vi "readArmPotValues.vi"(11 "set":bool) -> (3 "Normalized Value":dbl format="%#.5f")   [LabVIEW 2018]
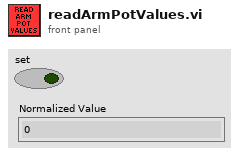
[diagram p1: front panel]
types:
  T1 = enum16{"open", "replace", "create", "open or create", "replace or create", "replace or create with confirmation"}
  T2 = typedef "WPI_PotentiometerDevRef.ctl" = cluster{"DevStatus":errorcluster, "Analog Channel":T3, "Invert Output":bool}
  T3 = typedef "FPGA_AIChannel.ctl" = enum8{"AI 0", "AI 1", "AI 2", "AI 3", "AI MXP 0", "AI MXP 1", "AI MXP 2", "AI MXP 3", "Invalid"}
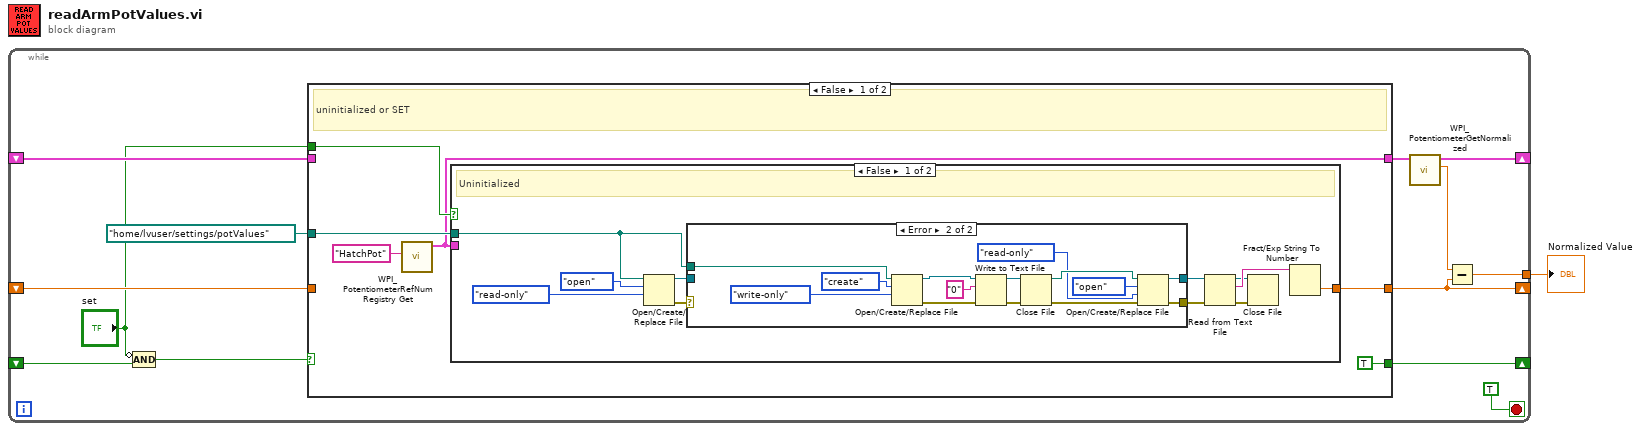
[diagram p0: block diagram]
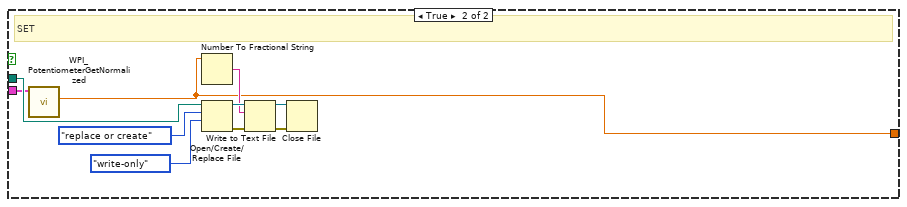
[diagram p3: hidden frame]
diagram:
  n1 = while {
    shift-right: [w14] -> _
    shift-left: _ -> [w13]
    shift-right: [w10] -> _
    shift-left: _ -> [w12]
    tunnel: [w7] -> w1
    shift-right: [w6] -> _
    shift-left: _ -> [w5]
    stop <- TRUE stop-if-true
    n2 = Compound Arithmetic op=AND(invert "set", w13) -> (w4:bool)
    n3 = case shown="False" w4 {
      selector: w4 -> [_ w60]
      tunnel: [TRUE w60] -> w14
      tunnel: [w15 w59] -> w11
      tunnel: w12 -> [_ w59]
      tunnel: [w18 w58] -> w6
      tunnel: w5 -> [_ w58]
      tunnel: "set" -> [w17 _]
      tunnel: path "/home/lvuser/settings/potValues" ("file path (use dialog)") -> [w16 _]
      frame False {
        # "uninitialized or SET"
        n4 = call <vilib>:"WPI_PotentiometerRefNum Registry Get.vi"("refnum name"="HatchPot") -> ("PotDevRef"=w15:T2)  [unwired: 9 in, 1 out]
        n5 = case shown="False" w17 {
          tunnel: [w24 w49] -> w18
          tunnel: w16 -> [w23 w50]
          tunnel: w15 -> [_ w48]
          frame False {
            # "Uninitialized"
            n6 = Open/Create/Replace File(file path (use dialog)=w23, operation (0:open)=T1."open", access (0:read/write)=enum16{"read/write", "read-only", "write-only"}."read-only") -> (refnum out=w28:refnum<file>, error out=w29:errorcluster)  [unwired: 3 in, 1 out]
            n7 = case shown="Error" w29 {
              selector: w29 -> [w33 _]
              tunnel: w28 -> [w32 _]
              tunnel: w23 -> [_ w47]
              tunnel: [w33 w34] -> w27
              tunnel: [w32 w35] -> w26
              frame No Error {
              }
              frame Error {
                n8 = Open/Create/Replace File(file path (use dialog)=w47, operation (0:open)=T1."create", access (0:read/write)=enum16{"read/write", "read-only", "write-only"}."write-only") -> (refnum out=w43:refnum<file>, error out=w44:errorcluster)  [unwired: 3 in, 1 out]
                n9 = Write to Text File(file (use dialog)=w43, text="0", error in=w44) -> (refnum out=w41:refnum<file>, error out=w40:errorcluster)  [unwired: 1 in, 1 out]
                n10 = Close File(refnum=w41, error in=w40) -> (path=w38:path, error out=w39:errorcluster)
                n11 = Open/Create/Replace File(file path (use dialog)=w38, error in=w39, operation (0:open)=T1."open", access (0:read/write)=enum16{"read/write", "read-only", "write-only"}."read-only") -> (refnum out=w35:refnum<file>, error out=w34:errorcluster)  [unwired: 2 in, 1 out]
              }
            }
            n12 = Read from Text File(file (use dialog)=w26, error in=w27) -> (refnum out=w21:refnum<file>, text=w25:string, error out=w22:errorcluster)  [unwired: 2 in, 1 out]
            n13 = Close File(refnum=w21, error in=w22) -> ()  [unwired: 2 out]
            n14 = Fract/Exp String To Number(string=w25) -> (number=w24:dbl)  [unwired: 3 in, 1 out]
          }
          frame True {
            # "SET"
            n15 = call <vilib>:"WPI_PotentiometerGetNormalized.vi"("PotDevRef"=w48) -> ("Normalized Value"=w49:dbl)  [unwired: 8 in, 2 out]
            n16 = Number To Fractional String(number=w49) -> (F-format string=w53:string)  [unwired: 3 in]
            n17 = Open/Create/Replace File(file path (use dialog)=w50, operation (0:open)=T1."replace or create", access (0:read/write)=enum16{"read/write", "read-only", "write-only"}."write-only") -> (refnum out=w54:refnum<file>, error out=w55:errorcluster)  [unwired: 3 in, 1 out]
            n18 = Write to Text File(file (use dialog)=w54, text=w53, error in=w55) -> (refnum out=w51:refnum<file>, error out=w52:errorcluster)  [unwired: 1 in, 1 out]
            n19 = Close File(refnum=w51, error in=w52) -> ()  [unwired: 2 out]
          }
        }
      }
      frame True {
      }
    }
    n20 = call <vilib>:"WPI_PotentiometerGetNormalized.vi"("PotDevRef"=w11) -> ("Normalized Value"=w9:dbl, "PotDevRef"=w10:T2)  [unwired: 8 in, 1 out]
    n21 = Subtract(x=w9, y=w6) -> (x-y=w7:dbl)
  }
  "Normalized Value" <- w1
